vi "AMZ_S3_APIHLP_Convert LocationConstraint Enum to String.vi"(4 "Location":T1) -> (1 "Location String":string)   [LabVIEW 2015, in "LV Interface for Amazon S3.lvlib"]
doc: "Convert the Bucket Location represented as a String to the Enum typedef representation."
uses:
  LV Interface for Amazon S3.lvlib
  Typedefs/AMZ_S3_LocationConstraint.ctl
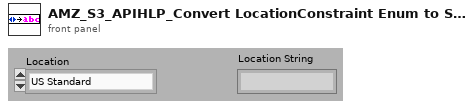
[diagram p1: front panel]
types:
  T1 = typedef "LV Interface for Amazon S3.lvlib/AMZ_S3_LocationConstraint.ctl" = enum16{"US Standard", "us-east-2", "us-west-1", "us-west-2", "ap-northeast-1", "ap-northeast-2", "ap-southeast-1", "ap-southeast-2", "ca-central-1", "eu-central-1", "eu-west-1", "eu-west-2", "sa-east-1"}
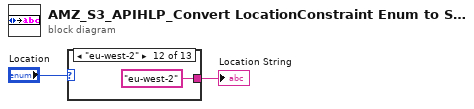
[diagram p0: block diagram]
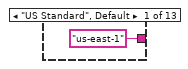
[diagram p2: hidden frame]
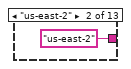
[diagram p3: hidden frame]
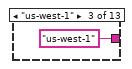
[diagram p4: hidden frame]
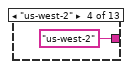
[diagram p5: hidden frame]
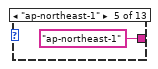
[diagram p6: hidden frame]
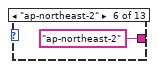
[diagram p7: hidden frame]
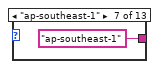
[diagram p8: hidden frame]
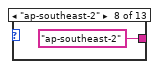
[diagram p9: hidden frame]
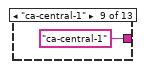
[diagram p10: hidden frame]
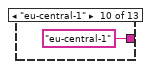
[diagram p11: hidden frame]
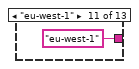
[diagram p12: hidden frame]
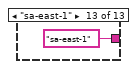
[diagram p13: hidden frame]
diagram:
  n1 = case shown="\"eu-west-2\"" "Location" {
    tunnel: ["us-east-1" "us-east-2" "us-west-1" "us-west-2" "ap-northeast-1" "ap-northeast-2" "ap-southeast-1" "ap-southeast-2" "ca-central-1" "eu-central-1" "eu-west-1" "eu-west-2" "sa-east-1"] -> w1
    frame "US Standard", Default {
    }
    frame "us-east-2" {
    }
    frame "us-west-1" {
    }
    frame "us-west-2" {
    }
    frame "ap-northeast-1" {
    }
    frame "ap-northeast-2" {
    }
    frame "ap-southeast-1" {
    }
    frame "ap-southeast-2" {
    }
    frame "ca-central-1" {
    }
    frame "eu-central-1" {
    }
    frame "eu-west-1" {
    }
    frame "eu-west-2" {
    }
    frame "sa-east-1" {
    }
  }
  "Location String" <- w1
